vi "Create channel error check (SubVI).vi"(8 "error in (no error)":errorcluster, 9 "Phisical channels":T3[](array[typedef]) items=["None", "AI1", "AI2", "AI3", "AI4", "AI5", "AI6", "AI7", "AI8", "AI9", "AI10", "AI11", "AI12", "AI13", "AI14", "AI15", "AI16"], 10 "Ranges":T2[](array[typedef]), 11 "Input terminals configurations":T1[](array[typedef])) -> (0 "error out":errorcluster)   [LabVIEW 2009, in "MicroDAQ.lvlib" / "Analog Input.lvclass"]
uses:
  <instrlib>/MicroDAQ/Channel/Analog Input/Analog Input.lvclass
  <instrlib>/MicroDAQ/Tools/Analog input Channel enum.ctl
  <instrlib>/MicroDAQ/Tools/Analo Range Enum.ctl
  <instrlib>/MicroDAQ/Tools/Analog input type enum.ctl
  <instrlib>/MicroDAQ/MicroDAQ.lvlib
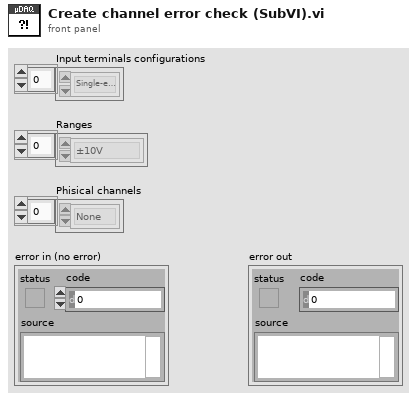
[diagram p1: front panel]
types:
  T1 = typedef "MicroDAQ.lvlib/Analog input type enum.ctl" = enum8{"Single-ended", "Differential"}
  T2 = typedef "MicroDAQ.lvlib/Analo Range Enum.ctl" = enum16{"±10V", "0-10V", "±5V", "0-5V", "±5.12V", "±2.56V", "±2.5V", "±2V", "±1.24V", "±0.64V"}
  T3 = typedef "MicroDAQ.lvlib/Analog input Channel enum.ctl" = u16
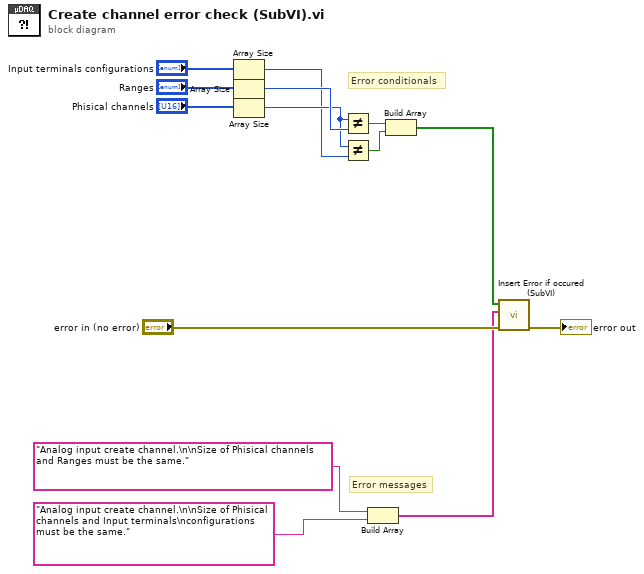
[diagram p0: block diagram]
diagram:
  # "Error messages"
  # "Error conditionals"
  n1 = Array Size(array="Input terminals configurations") -> (size(s)=w7:i32)
  n2 = Array Size(array="Ranges") -> (size(s)=w9:i32)
  n3 = Array Size(array="Phisical channels") -> (size(s)=w8:i32)
  n4 = Not Equal?(x=w8, y=w9) -> (x != y?=w6:bool)
  n5 = Not Equal?(x=w8, y=w7) -> (x != y?=w5:bool)
  n6 = Build Array("Analog input create channel.\n\nSize of Phisical channels and Ranges must be the same.", "Analog input create channel.\n\nSize of Phisical channels and Input terminals\nconfigurations must be the same.") -> (w1:string[])
  n7 = Build Array(w6, w5) -> (w2:bool[])
  n8 = call <instrlib>:"Insert Error if occured (SubVI).vi"("error in (no error)"="error in (no error)", "Error messages"=w1, "Error conditionals"=w2) -> ("error out"=→"error out":errorcluster)  [unwired: 8 in]
